vi "Thorlabs_TDC001.MoveAbsolute.vi"(0 "i ref in":refnum<vi>, 3 "fAbsPos in":sgl, 5 "error in (no error)":errorcluster) -> (14 "i ref out":refnum<vi>, 16 "fAbsPos out":sgl, 19 "error out":errorcluster)   [LabVIEW 2014, in "Thorlabs_TDC001.lvlib"]
doc: "This is the constructor of a class.\n\nLicense Agreement for this software:\n\nCopyright (C)\nGesellschaft für Schwerionenforschung, GSI\nPlanckstr. 1\n64291 Darmstadt\nGermany\n\nContact: D.Beck@gsi.de \n\nThis program is free software; you can redistribute it and/or modify it under the terms of the \nGNU General Public License as published by the Free Software Foundation; either version 2 of \nthe license, or (at your option) any later version.\n\nThis program is distributed in the hope that it will be useful, but WITHOUT ANY WARRANTY; \nwithout even the implied warranty of MERCHANTABILITY or FITNESS FOR A PARTICULAR PURPOSE. See the GNU General License for more details (http://www.gnu.org).\n\nGesellschaft für Schwerionenforschung, GSI\nPlanckstr. 1, 64291 Darmstadt, Germany\nFor all questions and ideas contact: M.Richter@gsi.de, H.Brand@gsi.de or D.Beck@gsi.de.\nLast update: 16-JUN-2004"
uses:
  Thorlabs_TDC001.lvlib
panel:
  in  "MG17Motor":refnum<k7>(container)
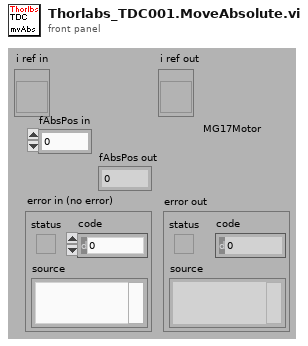
[diagram p1: front panel]
types:
  T1 = typedef "Thorlabs_TDC001.lvlib/Thorlabs_TDC001.i attribute.ctl" = cluster{"SerialNo":i32, "ChannelID":i32}
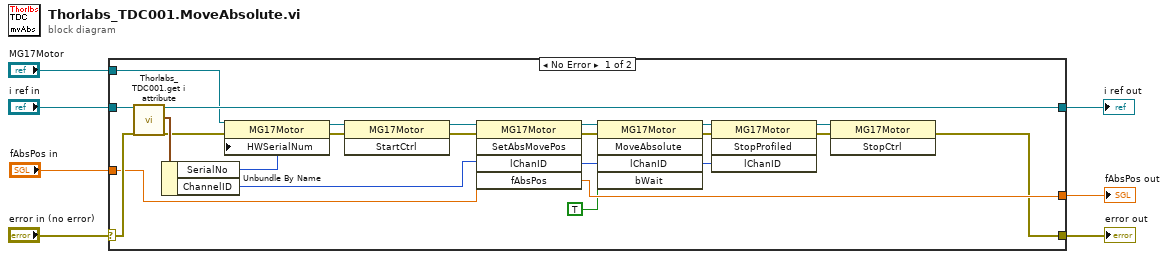
[diagram p0: block diagram]
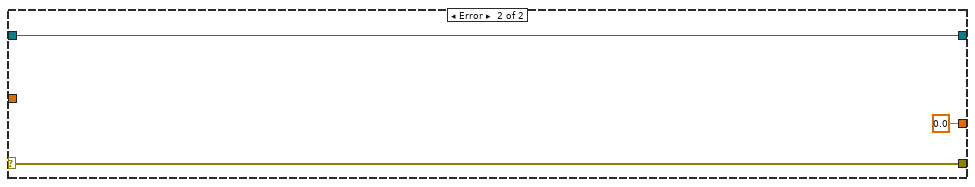
[diagram p2: hidden frame]
diagram:
  n1 = case shown="No Error" "error in (no error)" {
    selector: "error in (no error)" -> [w30 w34]
    tunnel: [w8 w34] -> w7
    tunnel: "i ref in" -> [w31 w33]
    tunnel: [w28 w33] -> w4
    tunnel: [w23 sgl 0.0 ("fAbsPos")] -> w3
    tunnel: "fAbsPos in" -> [w24 _]
    tunnel: "MG17Motor" -> [w16 _]
    frame No Error {
      n2 = call "Thorlabs_TDC001.get i attribute.vi"("i ref in"=w31, "error in (no error)"=w30) -> ("i ref out"=w28:refnum<vi>, "i attribute"=w29:T1, "error out"=w17:errorcluster)  [unwired: 15 in]
      n3 = Unbundle By Name(w29) -> ("SerialNo"=w11:i32, "ChannelID"=w18:i32)
      n4 = property class="MG17Motor"(reference=w16, error in=w17, "HWSerialNum"=w11) -> (reference out=w15:refnum<k7>, error out=w14:errorcluster)
      n5 = invoke class="MG17Motor" method="StartCtrl"(reference=w15, error in=w14) -> (reference out=w13:refnum<k7>, error out=w12:errorcluster)  [unwired: 1 in, 1 out]
      n6 = invoke class="MG17Motor" method="SetAbsMovePos"(reference=w13, error in=w12, "lChanID"=w18, "fAbsPos"=w24) -> (reference out=w27:refnum<k7>, error out=w26:errorcluster, "lChanID"=w25:i32, "fAbsPos"=w23:sgl)  [unwired: 1 in, 1 out]
      n7 = invoke class="MG17Motor" method="MoveAbsolute"(reference=w27, error in=w26, "lChanID"=w25, "bWait"=TRUE) -> (reference out=w21:refnum<k7>, error out=w20:errorcluster, "lChanID"=w19:i32)  [unwired: 1 in, 2 out]
      n8 = invoke class="MG17Motor" method="StopProfiled"(reference=w21, error in=w20, "lChanID"=w19) -> (reference out=w10:refnum<k7>, error out=w9:errorcluster)  [unwired: 1 in, 2 out]
      n9 = invoke class="MG17Motor" method="StopCtrl"(reference=w10, error in=w9) -> (error out=w8:errorcluster)  [unwired: 1 in, 2 out]
    }
    frame Error {
    }
  }
  "error out" <- w7
  "i ref out" <- w4
  "fAbsPos out" <- w3
